vi "Attenuator Convert Limits Cluster.vi"(5 "Conversion":enum16{"Cluster - HTML", "HTML - Cluster"}(ring), 7 "Limits Key Array In":T2, 8 "Limit Cluster In":T1) -> (1 "Limit Cluster Out":T1, 2 "Limits HTML Out":string)   [LabVIEW 2011]
uses:
  ITK EXT/utils/keyedarr.llb/Keyed Array.ctl
  TypeDefs/Attenuator Limit.ctl
  ITK EXT/utils/strutil.llb/Case Matching.ctl
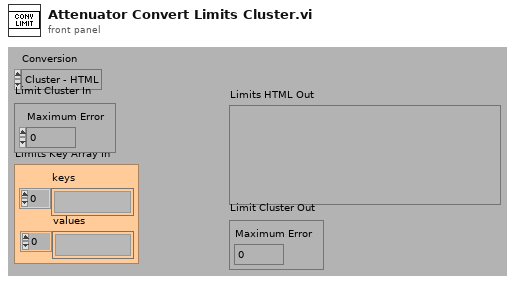
[diagram p1: front panel]
types:
  T1 = typedef "Attenuator Limit.ctl" = cluster{"Maximum Error":dbl}
  T2 = typedef "Keyed Array.ctl" = cluster{"keys":string[], "values":string[]}
  T3 = typedef "Case Matching.ctl" = enum16{"a != A", "a == A", "system"}
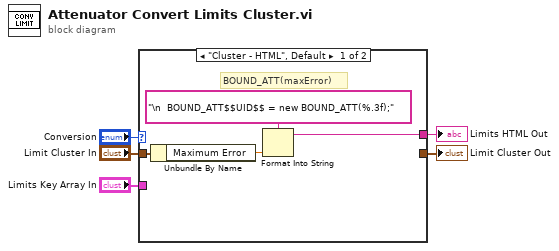
[diagram p0: block diagram]
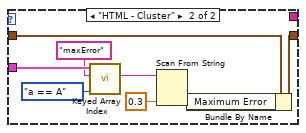
[diagram p2: hidden frame]
diagram:
  n1 = case shown="\"Cluster - HTML\", Default" "Conversion" {
    tunnel: "Limit Cluster In" -> [w7 w13]
    tunnel: "Limits Key Array In" -> [_ w17]
    tunnel: [w9 _] -> w2
    tunnel: [_ w14] -> w1
    frame "Cluster - HTML", Default {
      # "BOUND_ATT(maxError)"
      n2 = Unbundle By Name(w7) -> ("Maximum Error"=w6:dbl)
      n3 = Format Into String(format string="\n  BOUND_ATT$$UID$$ = new BOUND_ATT(%.3f);", w6) -> (resulting string=w9:string)  [unwired: 2 in, 1 out]
    }
    frame "HTML - Cluster" {
      n4 = call "Keyed Array Index.vi"("case matching (sensitive)"=Case_Matching."a == A", "key"="maxError", "array in"=w17) -> ("value"=w11:string)  [unwired: 1 in, 3 out]
      n5 = Scan From String(input string=w11, default 1=0.3 ("default value 1")) -> (output 1=w10:dbl)  [unwired: 3 in, 3 out]
      n6 = Bundle By Name(cluster=w13, "Maximum Error"=w10) -> (w14:T1)
    }
  }
  "Limits HTML Out" <- w2
  "Limit Cluster Out" <- w1
